vi "readsensor.vi"(1 "Y":i8, 2 "X":i8, 3 "World":i8[][](array[numeric])) -> (0 "Sensor Array":i8[][](array[numeric]))   [LabVIEW 2012]
doc: "This VI returns the 3x3 array that is visible to the robot when it is at a given location. It has safeguards in place to make sure it returns the correct data when the X,Y coordinate is on the edge of the world."
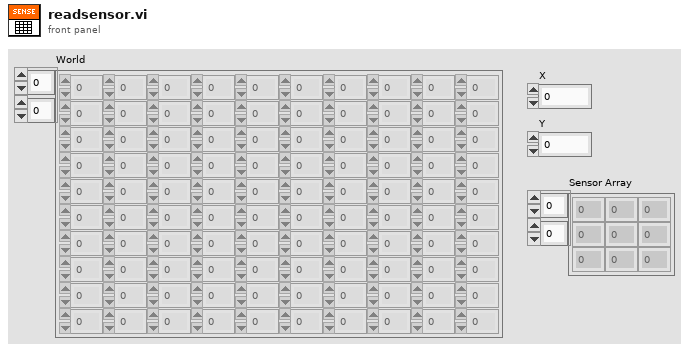
[diagram p1: front panel]
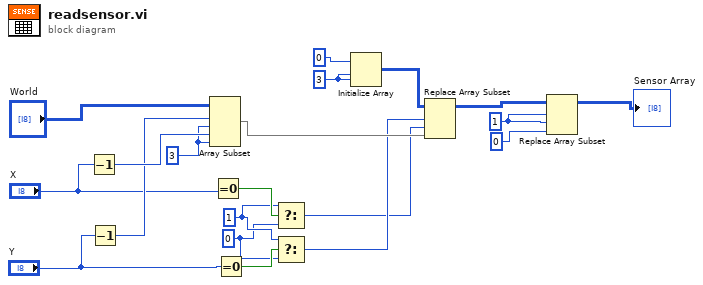
[diagram p0: block diagram]
diagram:
  w2 = 1
  w9 = 0
  w10 = 1
  w16 = 3
  w17 = 3
  n1 = Decrement(x="X") -> (x-1=w19:i8)
  n2 = Decrement(x="Y") -> (x-1=w18:i8)
  n3 = Array Subset(array="World", index (row)=w18, length (row)=w17, index (col)=w19, length (col)=w17) -> (w6:i8[][])
  n4 = Equal To 0?(x="X") -> (x = 0?=w11:bool)
  n5 = Equal To 0?(x="Y") -> (x = 0?=w12:bool)
  n6 = Select(t=w10, s=w11, f=w9) -> (s? t:f=w4:i32)
  n7 = Select(t=w10, s=w12, f=w9) -> (s? t:f=w5:i32)
  n8 = Initialize Array(i8 0, w16, w16) -> (w7:i8[][])
  n9 = Replace Array Subset(array=w7, new element=w6, index (row)=w5, index (col)=w4) -> (w8:i8[][])
  n10 = Replace Array Subset(array=w8, new element=i8 0, index (row)=w2, index (col)=w2) -> (→"Sensor Array":i8[][])
